vi "Convert 12bit ADC to kg.vi"(10 "ADC":i16) -> (2 "output":dbl)   [LabVIEW 2011]
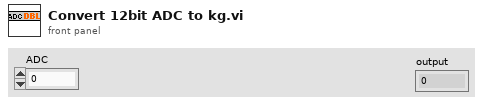
[diagram p1: front panel]
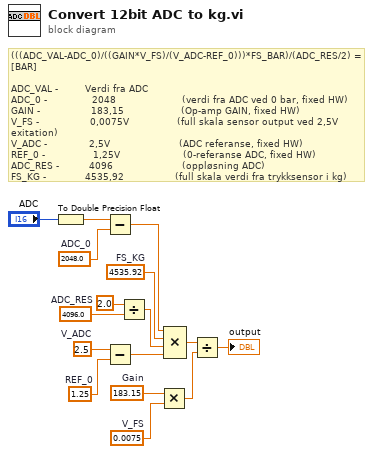
[diagram p0: block diagram]
diagram:
  w10 = 4096.0  # ADC_RES
  w8 = 4535.92  # FS_KG
  w12 = 1.25  # REF_0
  w13 = 2.5  # V_ADC
  w14 = 0.0075  # V_FS
  w15 = 183.15  # Gain
  w16 = 2048.0  # ADC_0
  # "(((ADC_VAL-ADC_0)/((GAIN*V_FS)/(V_ADC-REF_0)))*FS_BAR)/(ADC_RES/2) = [BAR]\n\nADC_VAL -         Verdi fra ADC\nADC_0 -               2048                      (verdi fra ADC ved 0 bar, fixed HW)\nGAIN -                 183,15                   (Op-amp GAIN, fixed HW)\nV_FS -                 0,0075V                (full skala sensor output ved 2,5V exitation)\nV_ADC -              2,5V                       (ADC referanse, fixed HW)\nREF_0 -                1,25V                     (0-referanse ADC, fixed HW)\nADC_RES -          4096                       (oppløsning ADC)\nFS_KG -             4535,92                 (full skala verdi fra trykksensor i kg)"
  n1 = To Double Precision Float(number="ADC") -> (double precision float=w1:dbl)
  n2 = Subtract(x=w1, y=w16) -> (x-y=w9:dbl)
  n3 = Subtract(x=w13, y=w12) -> (x-y=w6:dbl)
  n4 = Divide(x=2.0, y=w10) -> (x/y=w7:dbl)
  n5 = Multiply(x=w15, y=w14) -> (x*y=w4:dbl)
  n6 = Compound Arithmetic op=MULTIPLY(w9, w8, w7, w6) -> (w5:dbl)
  n7 = Divide(x=w5, y=w4) -> (x/y=→"output":dbl)
